vi "Plotter parse device data.vi"(11 "ShotData":string[](array[string])) -> (2 "Shot #":string, 3 "Shot Data parsed array":string[][](array[string]))   [LabVIEW 2009]
uses:
  <userlib>/_OpenG.lib/array/array.llb/Delete Elements from 1D Array (String)__ogtk.vi
  <userlib>/_OpenG.lib/array/array.llb/Search 1D Array (String)__ogtk.vi
panel:
  in  "delete ones":bool=TRUE
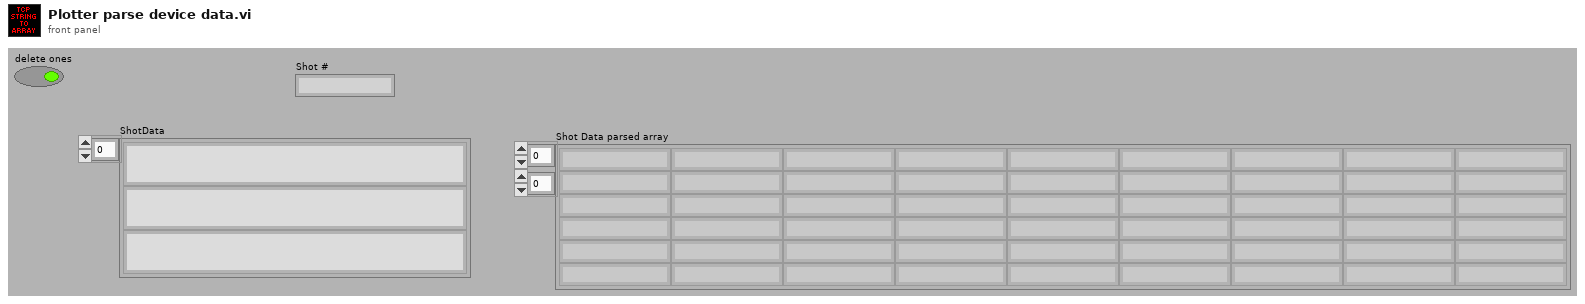
[diagram p1: front panel]
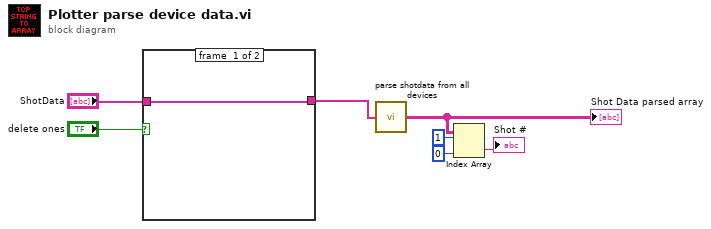
[diagram p0: block diagram]
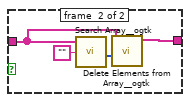
[diagram p2: hidden frame]
diagram:
  n1 = case shown="True" "delete ones" {
    tunnel: "ShotData" -> [w8 w10]
    tunnel: [w8 w9] -> w6
    frame #0 {
    }
    frame #1 {
      n2 = call-poly <userlib>:"Search Array__ogtk.vi"("Array"=w10, "Element Data"="") -> ("Indices of Elements"=w11:i32[])  [unwired: 7 in]
      n3 = call-poly <userlib>:"Delete Elements from Array__ogtk.vi"("indices"=w11, "array"=w10) -> ("array w/ subset deleted"=w9:string[])  [unwired: 8 in, 1 out]
    }
  }
  n4 = call "parse shotdata from all devices.vi"("ShotData"=w6) -> ("Shot Data parsed array"=w5:string[][])
  "Shot Data parsed array" <- w5
  n5 = Index Array(array=w5, index (row)=1 ("disabled index (row)"), index (col)=0 ("disabled index (col)")) -> (element=→"Shot #":string)
